vi "GetAllPaths.vi"(0 "LocalName":string) -> (1 "Hard Path":path, 2 "Top Level":path, 3 "User Documents":path)   [LabVIEW 2015]
doc: "Gets the paths for LVROS, the servers, _BlankServer, and the Master Console"
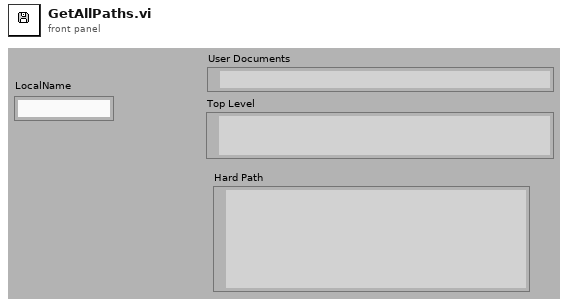
[diagram p1: front panel]
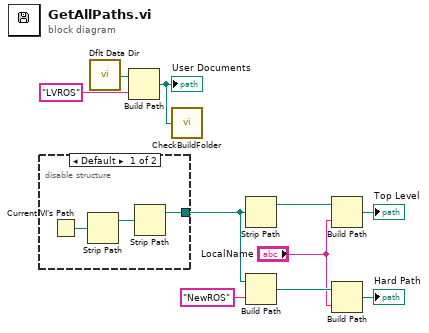
[diagram p0: block diagram]
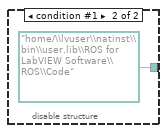
[diagram p2: hidden frame]
diagram:
  n1 = disable-structure shown="Default" {
    disable-tunnel: [w11 path "/home/\\lvuser\\natinst\\bin\\user.lib\\ROS for LabVIEW Software\\ROS\\Code" ("stripped path")] -> w4
    frame condition #0 (active) {
      n2 = Current VI's Path() -> (path=w12:path)
      n3 = Strip Path(path=w12) -> (stripped path=w13:path)  [unwired: 1 out]
      n4 = Strip Path(path=w13) -> (stripped path=w11:path)  [unwired: 1 out]
    }
    frame condition #1 {
    }
  }
  n5 = call "Dflt Data Dir.vi"() -> ("App:Default Data Directory"=w9:path)
  n6 = Build Path(base path=w9, name or relative path="LVROS") -> (appended path=w8:path)
  "User Documents" <- w8
  n7 = call "CheckBuildFolder.vi"("appended path"=w8) -> ()  [unwired: 1 in]
  n8 = Strip Path(path=w4) -> (stripped path=w3:path)  [unwired: 1 out]
  n9 = Build Path(base path=w4, name or relative path="NewROS") -> (appended path=w7:path)
  n10 = Build Path(base path=w3, name or relative path="LocalName") -> (appended path=→"Top Level":path)
  n11 = Build Path(base path=w7, name or relative path="LocalName") -> (appended path=→"Hard Path":path)
